vi "CreatePublicEvents.vi"(8 "error in (no error)":errorcluster, 11 "Instrument.Lockin":refnum<class "Instrument.Lockin.lvclass">) -> (0 "error out":errorcluster, 3 "Instrument.Lockin out":refnum<class "Instrument.Lockin.lvclass">)   [LabVIEW 2019, in "Instrument.Lockin.lvclass"]
doc: "---------------------------------------------------------------\nJKI State Machine Objects™\nhttp://jki.net/state-machine-objects/\nCopyright (C) 2005-2015, JKI <info@jki.net>\nALL RIGHTS RESERVEDJKI State Machine Objects (SMO) 1.0.0.4\nJKI - JKI\nCopyright (c) 2015, JKI"
uses:
  Instrument.Lockin.lvclass
  <userlib>/LevyLab/Instrument Framework/SMOs/Instrument/Instrument.lvclass
  Typedefs/PublicEvents--Instrument.Lockin.getAO.ctl
panel:
  # "For instructions on how to use the JKI State Machine Objects, examples and video tutorials, visit:\nhttp://jki.net/state-machine-objects/\n\nJKI State Machine Objects™\nhttp://jki.net/state-machine-objects/\nCopyright (C) 2005-2015, JKI <info@jki.net>\nALL RIGHTS RESERVED"
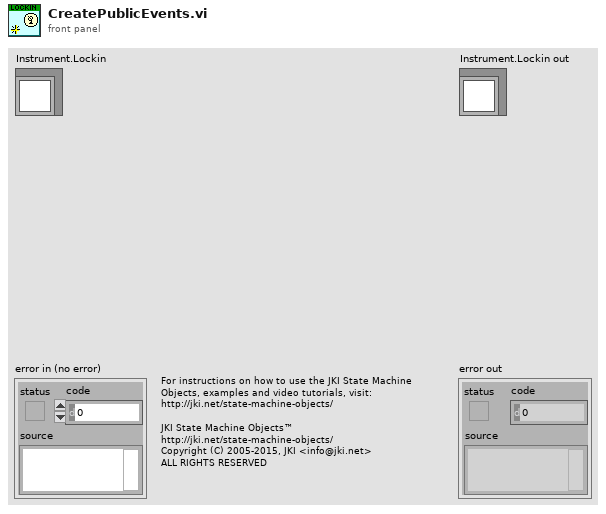
[diagram p1: front panel]
types:
  T1 = typedef "Instrument.Lockin.lvclass/PublicEvents--Instrument.Lockin.getAO.ctl" = waveform(dbl)[]
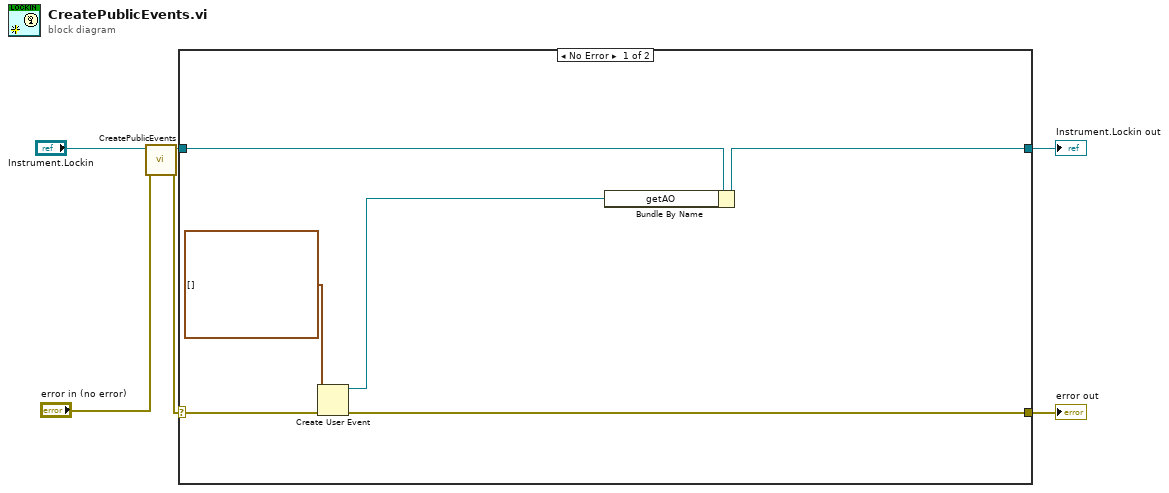
[diagram p0: block diagram]
diagram:
  n1 = call-parent "CreatePublicEvents.vi"("error in (no error)"="error in (no error)", "Instrument"="Instrument.Lockin") -> ("error out"=w3:errorcluster, "Instrument out"=w4:refnum<class "Instrument.Lockin.lvclass">)  [unwired: 8 in]
  n2 = case shown="No Error" w3 {
    selector: w3 -> [w11 w14]
    tunnel: [w9 w14] -> w5
    tunnel: [w10 w13] -> w1
    tunnel: w4 -> [w12 w13]
    frame No Error {
      n3 = Create User Event(user event datatype=T1 [] ("getAO"), error in=w11) -> (user event=w7:refnum<user-event>, error out=w9:errorcluster)
      n4 = Bundle By Name(cluster=w12, "getAO"=w7) -> (w10:refnum<class "Instrument.Lockin.lvclass">)
    }
    frame Error {
    }
  }
  "error out" <- w5
  "Instrument.Lockin out" <- w1
